vi "Draw Filled Triangle 1D.vi"(10 "Triangle":T1={"Vertex 1"={"Position"={"x"=0.0, "y"=0.0, "z"=0.0}, "UV"={"u"=0.0, "v"=0.0}, "Colour"=12517256}, "Vertex 2"={"Position"={"x"=0.0, "y"=0.0, "z"=0.0}, "UV"={"u"=0.0, "v"=0.0}, "Colour"=12517256}, "Vertex 3"={"Position"={"x"=0.0, "y"=0.0, "z"=0.0}, "UV"={"u"=0.0, "v"=0.0}, "Colour"=12517256}, "Alpha"=0.0, "Alpha Blending Enabled"=FALSE, "Colour"=0, "Material"={"Diffuse Colour"=0, "Texture"={"Pixels"=refnum, "Size"={"Width"=0, "Height"=0}}}} {"Vertex 3"."UV"."v" min=0 max=1 step=0.1; "Vertex 3"."UV"."u" min=0 max=1 step=0.1; "Vertex 2"."UV"."v" min=0 max=1 step=0.1; "Vertex 2"."UV"."u" min=0 max=1 step=0.1; "Vertex 1"."UV"."v" min=0 max=1 step=0.1; "Vertex 1"."UV"."u" min=0 max=1 step=0.1}, 11 "Pixel Data in":u32[](array[numeric])) -> (3 "Pixel Data out":u32[](array[numeric]))   [LabVIEW 2020, in "Raster (FPGA).lvlib"]
uses:
  Raster (FPGA).lvlib
  Libraries/Utility/Utility.lvlib
  Global 1.vi
  3D/3D (FPGA).lvlib
  UV.ctl
  <vilib>/Utility/miscctls.llb/LVPointTypeDef.ctl
  3D/Vector 3D.ctl
  3D/Vertex.ctl
  3D/Triangle.ctl
  Rectangle Dimensions.ctl
  Texture.ctl
  3D/Material.ctl
panel:
  out "Top Vertex.Colour":u32(colorbox)
  out "new picture":picture
  in  "Zoom Factor":sgl=5.0
  in  "Origin":T8={"Horizontal"=0, "Vertical"=426}
  # "(0,1)"
  # "(1,1)"
  # "(0,0)"
  # "(1,0)"
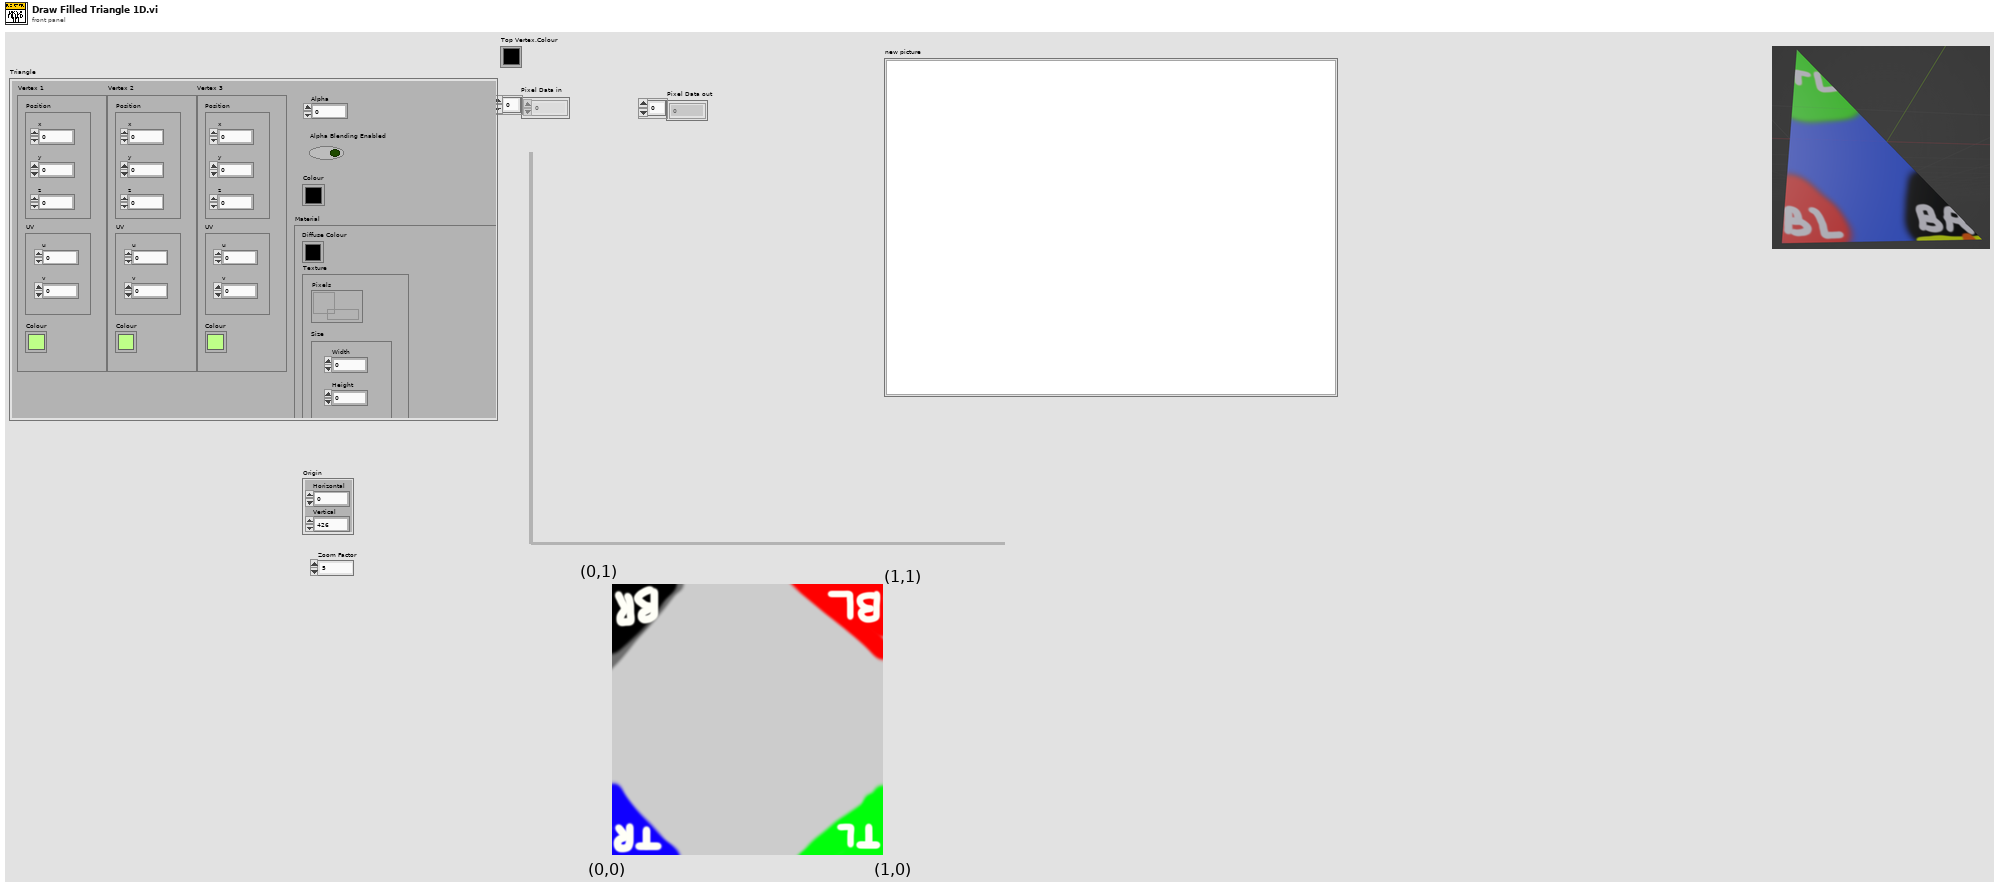
[diagram p1: front panel]
types:
  T1 = typedef "3D (FPGA).lvlib/Triangle.ctl" = cluster{"Vertex 1":T2, "Vertex 2":T2, "Vertex 3":T2, "Alpha":dbl, "Alpha Blending Enabled":bool, "Colour":u32, "Material":T5}
  T2 = typedef "3D (FPGA).lvlib/Vertex.ctl" = cluster{"Position":T3, "UV":T4, "Colour":u32}
  T3 = typedef "3D (FPGA).lvlib/Vector 3D.ctl" = cluster{"x":sgl, "y":sgl, "z":sgl}
  T4 = typedef "Raster (FPGA).lvlib/UV.ctl" = cluster{"u":sgl, "v":sgl}
  T5 = typedef "3D (FPGA).lvlib/Material.ctl" = cluster{"Diffuse Colour":u32, "Texture":T6}
  T6 = typedef "Raster (FPGA).lvlib/Texture.ctl" = cluster{"Pixels":refnum<data-value>, "Size":T7}
  T7 = typedef "Raster (FPGA).lvlib/Rectangle Dimensions.ctl" = cluster{"Width":u32, "Height":u32}
  T8 = typedef "LVPointTypeDef.ctl" = cluster{"Horizontal":i16, "Vertical":i16}
  T9 = typedef "3D (FPGA).lvlib/Triangle (Sorted).ctl" = cluster{"Top Vertex":T2, "Mid Vertex":T2, "Bottom Vertex":T2, "Alpha":dbl, "Alpha Blending Enabled":bool, "Colour":u32, "Material":T5}
  T10 = typedef "Raster (FPGA).lvlib/Reciprocals.ctl" = cluster{"Bottom --> Top":sgl, "Bottom --> Middle":sgl, "Middle --> Top":sgl}
  T11 = typedef "Raster (FPGA).lvlib/Current Row.ctl" = cluster{"Start Column":sgl, "End Column":sgl}
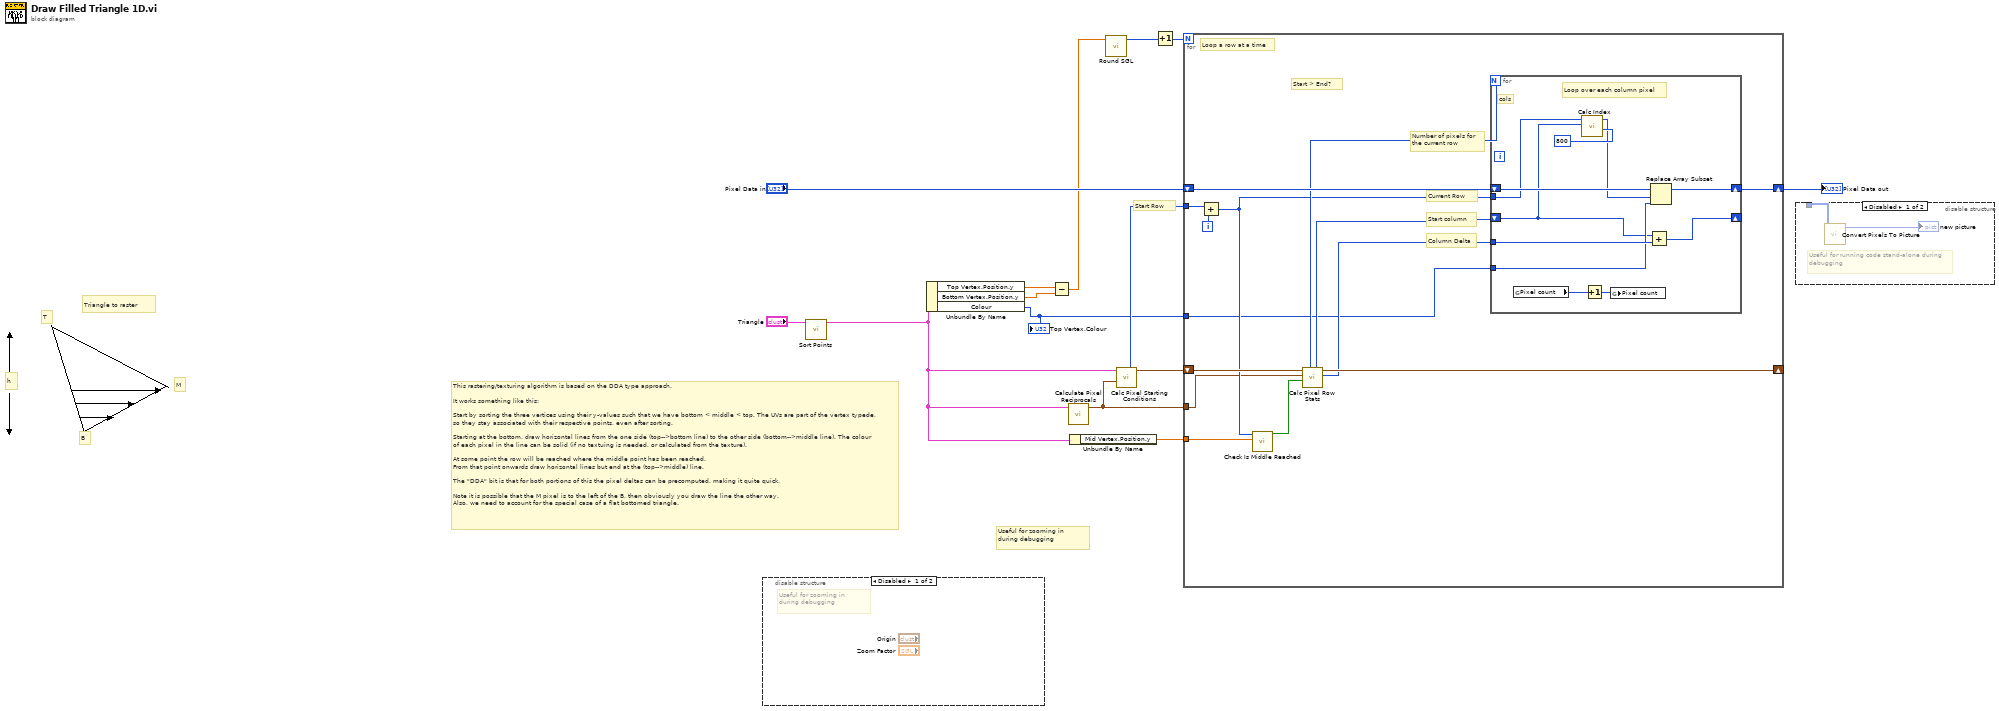
[diagram p0: block diagram]
diagram:
  # "h"
  # "Triangle to raster"
  # "M"
  # "T"
  # "B"
  # "This rastering/texturing algorithm is based on the DDA type approach.\n\nIt works something like this:\n\nStart by sorting the three vertices using their y-values such that we have bottom < middle < top. The UVs are part of the vertex typede, so they stay associated with their respective points, even after sorting.\n\nStarting at the bottom, draw horizontal lines from the one side (top-->bottom line) to the other side (bottom-->middle line). The colour of each pixel in the line can be solid (if no textuing is needed, or calculated from the texture).\n\nAt some point the row will be reached where the middle point has been reached.\nFrom that point onwards draw horizontal lines but end at the (top-->middle) line.\n\nThe \"DDA\" bit is that for both portions of this the pixel deltas can be precomputed, making it quite quick.\n\nNote it is possible that the M pixel is to the left of the B, then obviously you draw the line the other way.\nAlso, we need to account for the special case of a flat bottomed triangle."
  # "Useful for zooming in during debugging"
  # "Start Row"
  n1 = disable-structure shown="Disabled" {
    frame Disabled {
      # "Useful for zooming in during debugging"
    }
    frame Enabled {
    }
  }
  n2 = call "Sort Points.vi"("Triangle"="Triangle") -> ("Sorted Triangle"=w4:T9)  [unwired: 10 in]
  n3 = Unbundle By Name(w4) -> ("Top Vertex.Position.y"=w8:sgl, "Bottom Vertex.Position.y"=w7:sgl, "Colour"=w3:u32)
  "Top Vertex.Colour" <- w3
  n4 = Subtract(x=w8, y=w7) -> (x-y=w2:sgl)
  n5 = call "Calculate Pixel Reciprocals.vi"("Sorted Triangle"=w4) -> ("Columns Pixels Per Row"=w12:T10)  [unwired: 10 in]
  n6 = Unbundle By Name(w4) -> ("Mid Vertex.Position.y"=w6:sgl)
  n7 = call "Round SGL.vi"("SGL"=w2) -> ("I32"=w1:i32)  [unwired: 10 in]
  n8 = call "Calc Pixel Starting Conditions.vi"("Reciprocals"=w12, "Sorted Vertices (V1 is top)"=w4) -> ("Start Row Columns"=w13:T11, "Start Row"=w14:i32)  [unwired: 8 in]
  n9 = Increment(x=w1) -> (x+1=w10:i32)
  n10 = for {
    N: w10 -> [_]
    shift-right: [w29] -> w9
    shift-left: "Pixel Data in" -> [w30]
    tunnel: w14 -> [w28]
    shift-right: [w24] -> _
    shift-left: w13 -> [w26]
    tunnel: w6 -> [w22]
    tunnel: w12 -> [w21]
    tunnel: w3 -> [w17]
    i -> [w27]
    # "Column Delta"
    # "Start > End?"
    # "Current Row"
    # "Start column"
    # "Loop a row at a time"
    # "Number of pixels for the current row"
    n11 = Add(x=w28, y=w27) -> (x+y=w23:i32)
    n12 = call "Check Is Middle Reached.vi"("Middle y"=w22, "Current Row"=w23) -> ("Reached Middle"=w20:bool)  [unwired: 9 in]
    n13 = call "Calc Pixel Row Stats.vi"("Reached Middle"=w20, "Reciprocals"=w21, "Current Row"=w26) -> ("Column Delta"=w19:i32, "Next Row"=w24:T11, "Start Col"=w18:i32, "Number Of Cols This Row"=w25:i32)  [unwired: 4 in, 1 out]
    n14 = for {
      N: w25 -> [_]
      shift-right: [w38] -> w29
      shift-left: w30 -> [w39]
      tunnel: w23 -> [w33]
      shift-right: [w41] -> _
      shift-left: w18 -> [w32]
      tunnel: w19 -> [w40]
      tunnel: w17 -> [w37]
      # "Loop over each column pixel"
      # "cols"
      n15 = global read "Global 1.vi" "Pixel count"() -> (w36:u32)
      n16 = call "Calc Index.vi"("Cols Per Row"=800, "Col"=w32, "Row"=w33) -> ("Index"=w31:i32)  [unwired: 8 in]
      n17 = Increment(x=w36) -> (x+1=w35:u32)
      n18 = global write "Global 1.vi" "Pixel count"(w35) -> ()
      n19 = Add(x=w32, y=w40) -> (x+y=w41:i32)
      n20 = Replace Array Subset(array=w39, new element=w37, index=w31) -> (w38:u32[])
    }
  }
  "Pixel Data out" <- w9
  n21 = disable-structure shown="Disabled" {
    disable-tunnel: _ -> [w42 _]
    frame Disabled {
      # "Useful for running code stand-alone during debugging"
      n22 = call "Convert Pixels To Picture.vi"("Pixel Data in"=w42) -> ("2D Picture"=→"new picture":picture)  [unwired: 9 in, 1 out]
    }
    frame Enabled {
    }
  }
